vi "Test TCRS Temperature At Initial Value if Heater Disabled.vi"(8 "error in (no error)":errorcluster, 11 "Thermal Chamber Response Simlator Test In":refnum<class "Thermal Chamber Response Simlator Test.lvclass">) -> (0 "error out":errorcluster, 3 "Thermal Chamber Response Simlator Test Out":refnum<class "Thermal Chamber Response Simlator Test.lvclass">)   [LabVIEW 2020, in "Thermal Chamber Response Simlator Test.lvclass"]
uses:
  Thermal Chamber Response Simlator Test.lvclass
  Thermal Chamber Response Simlator/Thermal Chamber Response Simlator.lvclass
  <vilib>/Asteme/LUnit/Test Case.lvclass
  C:/Program Files (x86)/National Instruments/LabVIEW 2020/vi.lib/Asteme/LUnit/Test Case.lvclass
  C:/Users/anton/Documents/GitHub/Triarc-Examples/Thermal Chamber/Thermal Chamber Response Simlator Test/Thermal Chamber Response Simlator Test.lvclass
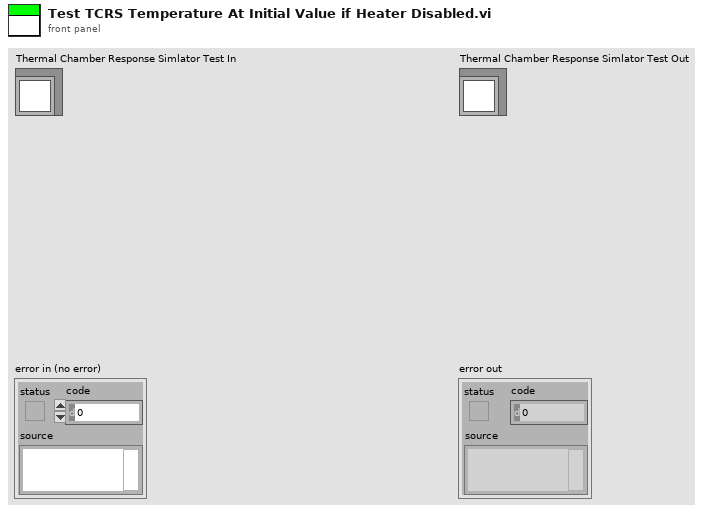
[diagram p1: front panel]
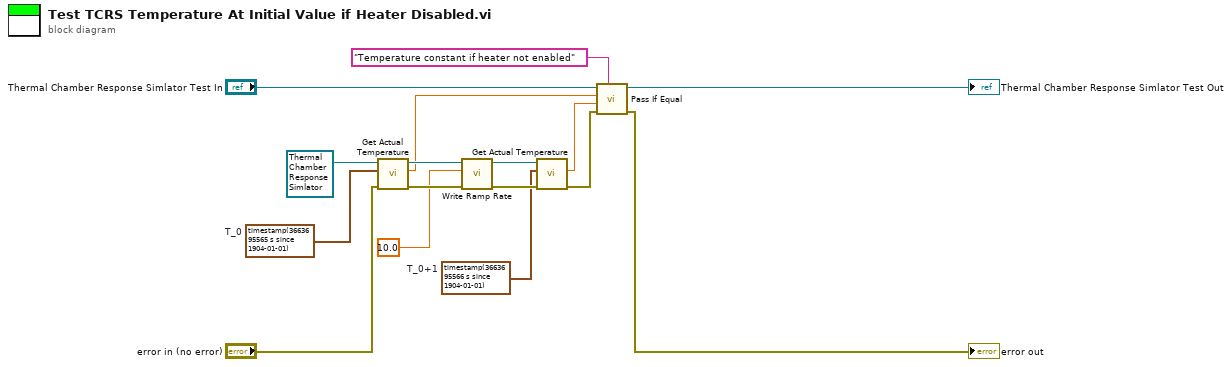
[diagram p0: block diagram]
diagram:
  w8 = timestamp(3663695566 s since 1904-01-01)  # T_0+1
  w14 = timestamp(3663695565 s since 1904-01-01)  # T_0
  n1 = call "Get Actual Temperature.vi"("error in (no error)"="error in (no error)", "Time Stamp"=w14, "Thermal Chamber Response Simlator In"=refnum<class "Thermal Chamber Response Simlator.lvclass"> refnum ("Thermal Chamber Response Simlator.lvclass")) -> ("error out"=w12:errorcluster, "Actual Temperature [degC]"=w4:dbl, "Thermal Chamber Response Simlator Out"=w13:refnum<class "Thermal Chamber Response Simlator.lvclass">)  [unwired: 6 in]
  n2 = call "Write Ramp Rate.vi"("error in (no error)"=w12, "Ramp Rate [degC/s]"=10.0, "Thermal Chamber Response Simlator In"=w13) -> ("error out"=w9:errorcluster, "Thermal Chamber Response Simlator Out"=w10:refnum<class "Thermal Chamber Response Simlator.lvclass">)  [unwired: 7 in]
  n3 = call "Get Actual Temperature.vi"("error in (no error)"=w9, "Time Stamp"=w8, "Thermal Chamber Response Simlator In"=w10) -> ("error out"=w6:errorcluster, "Actual Temperature [degC]"=w5:dbl)  [unwired: 6 in, 1 out]
  n4 = call <vilib>:"Pass If Equal.vi"("Description"="Temperature constant if heater not enabled", "error in (no error)"=w6, "Actual"=w5, "Expected"=w4, "Test Case In"="Thermal Chamber Response Simlator Test In") -> ("error out"=→"error out":errorcluster, "Test Case Out"=→"Thermal Chamber Response Simlator Test Out":refnum<class "Thermal Chamber Response Simlator Test.lvclass">)  [unwired: 5 in]
